vi "draw.vi"(0 "reference":refnum<class "ArrowHead.lvclass">, 1 "graphics":refnum<class "Graphics.lvclass">, 2 "p1":T1 {"y" format="%.2f"; "x" format="%.2f"}, 3 "p2":T1 {"y" format="%.2f"; "x" format="%.2f"}, 5 "error in (no error)":errorcluster) -> (14 "reference out":refnum<class "ArrowHead.lvclass">, 19 "error out":errorcluster)   [LabVIEW 2012, in "ArrowHead.lvclass"]
doc: "public void draw(Graphics2D g2, Point2D p, Point2D q)"
uses:
  <resource>/Framework/Providers/Open_GDS/UML/ArrowHead_class/ArrowHead.lvclass
  <resource>/Framework/Providers/Open_GDS/UML/Graphics_class/Graphics.lvclass
  <resource>/Framework/Providers/Open_GDS/UML/General/Point/Point Point2D.ctl
  <resource>/Framework/Providers/Open_GDS/UML/ArrowHead_class/ArrowHead.lvclass/ArrowHead.ctl
  <resource>/Framework/Providers/Open_GDS/UML/ArrowHead_class/ArrowHeadType.ctl
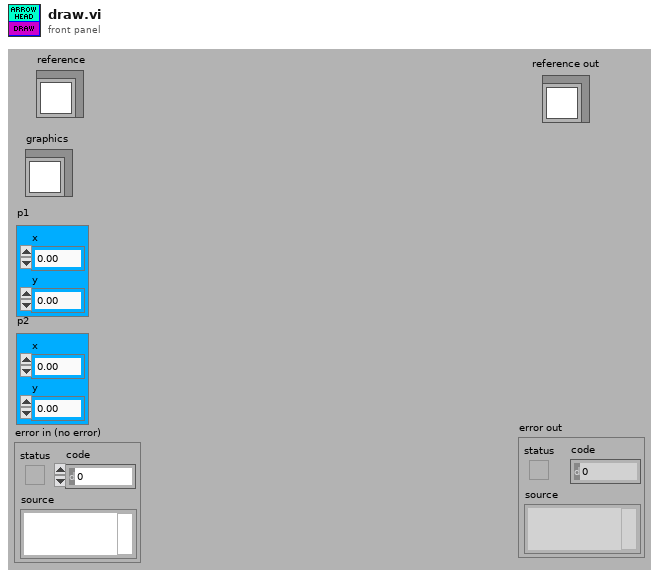
[diagram p1: front panel]
types:
  T1 = typedef "Point Point2D.ctl" = cluster{"x":dbl, "y":dbl}
  T2 = typedef "ArrowHead.lvclass/ArrowHeadType.ctl" = enum16{"NONE", "TRIANGLE", "BLACK_TRIANGLE", "V", "HALF_V", "DIAMOND", "BLACK_DIAMOND"}
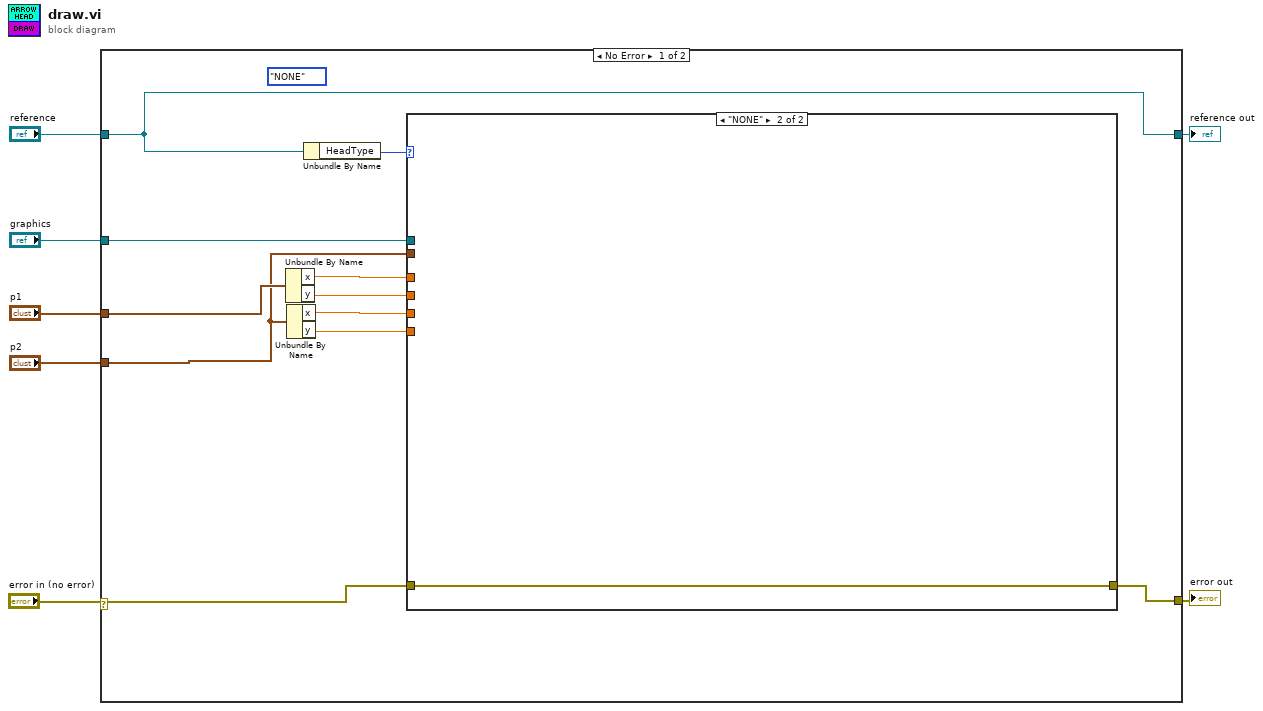
[diagram p0: block diagram]
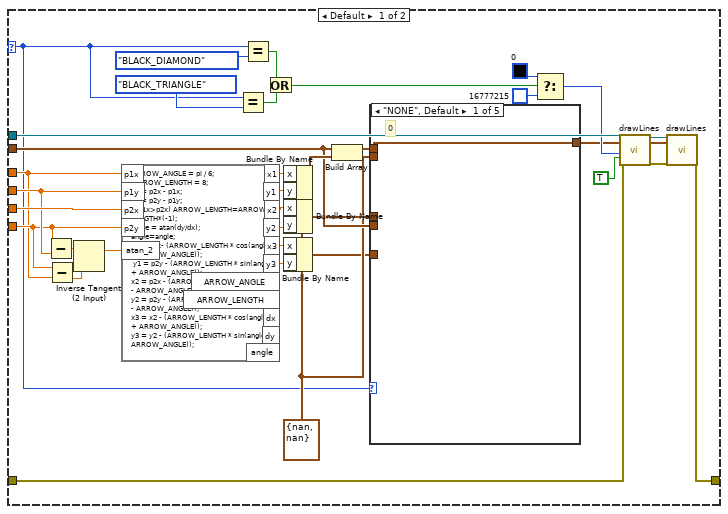
[diagram p2: hidden frame]
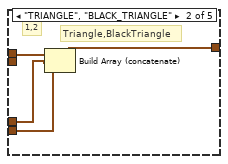
[diagram p3: hidden frame]
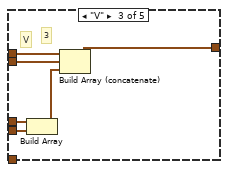
[diagram p4: hidden frame]
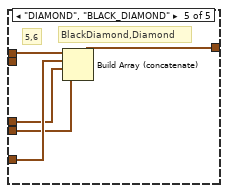
[diagram p6: hidden frame]
diagram:
  n1 = case shown="No Error" "error in (no error)" {
    selector: "error in (no error)" -> [w9 w72]
    tunnel: "reference" -> [w8 w73]
    tunnel: [w18 w72] -> w6
    tunnel: [w8 w73] -> w5
    tunnel: "graphics" -> [w17 _]
    tunnel: "p1" -> [w16 _]
    tunnel: "p2" -> [w15 _]
    frame No Error {
      (unwired) ArrowHeadType."NONE" ("HeadType")
      n2 = Unbundle By Name(w16) -> ("x"=w14:dbl, "y"=w13:dbl)
      n3 = Unbundle By Name(w15) -> ("x"=w12:dbl, "y"=w11:dbl)
      n4 = Unbundle By Name(w8) -> ("HeadType"=w10:T2)
      n5 = case shown="\"NONE\"" w10 {
        selector: w10 -> [w19 _]
        tunnel: w9 -> [w43 w71]
        tunnel: [w23 w71] -> w18
        tunnel: w17 -> [w53 _]
        tunnel: w14 -> [w27 _]
        tunnel: w13 -> [w30 _]
        tunnel: w12 -> [w47 _]
        tunnel: w11 -> [w28 _]
        tunnel: w15 -> [w39 _]
        frame Default {
          w37 = T1 {"x"=nan, "y"=nan} ("p1")
          n6 = Subtract(x=w28, y=w30) -> (x-y=w31:dbl)
          n7 = Subtract(x=w28, y=w27) -> (x-y=w29:dbl)
          n8 = Inverse Tangent (2 Input)(1:w29, 2:w31) -> (0:w32:dbl)
          n9 = formula code="ARROW_ANGLE = pi / 6;\n ARROW_LENGTH = 8;\ndx = p2x - p1x;\ndy = p2y - p1y;\nif(p1x>p2x) ARROW_LENGTH=ARROW_LENGTH*(-1);\nangle = atan(dy/dx);\nangle=angle;\nx1 = p2x- (ARROW_LENGTH * cos(angle + ARROW_ANGLE));\n y1 = p2y - (ARROW_LENGTH * sin(angle + ARROW_ANGLE));\nx2 = p2x - (ARROW_LENGTH * cos(angle - ARROW_ANGLE));\ny2 = p2y - (ARROW_LENGTH * sin(angle - ARROW_ANGLE));\nx3 = x2 - (ARROW_LENGTH * cos(angle + ARROW_ANGLE));\ny3 = y2 - (ARROW_LENGTH * sin(angle + ARROW_ANGLE));"("p1x"=w27, "p1y"=w30, "p2x"=w47, "p2y"=w28, "atan_2"=w32) -> ("x1"=w46:dbl, "y1"=w45:dbl, "x2"=w41:dbl, "y2"=w40:dbl, "x3"=w36:dbl, "y3"=w35:dbl)  [unwired: 5 out]
          n10 = Equal?(x=w19, y=ArrowHeadType."BLACK_TRIANGLE") -> (x = y?=w49:bool)
          n11 = Equal?(x=w19, y=ArrowHeadType."BLACK_DIAMOND") -> (x = y?=w21:bool)
          n12 = Or(x=w21, y=w49) -> (x .or. y?=w33:bool)
          n13 = Bundle By Name(cluster=w37, "x"=w46, "y"=w45) -> (w44:T1)
          n14 = Bundle By Name(cluster=w37, "x"=w41, "y"=w40) -> (w38:T1)
          n15 = Bundle By Name(cluster=w37, "x"=w36, "y"=w35) -> (w34:T1)
          n16 = Build Array(w39, w44) -> (w42:T1[])
          n17 = case shown="\"NONE\", Default" w19 {
            tunnel: w42 -> [w54 w58 w64 w65 w70]
            tunnel: w37 -> [_ _ w63 _ _]
            tunnel: w38 -> [_ w57 w61 _ w68]
            tunnel: w39 -> [_ w55 w60 _ w66]
            tunnel: w34 -> [_ _ _ _ w69]
            tunnel: [w54 w56 w59 w65 w67] -> w25
            frame "NONE", Default {
              # "0"
            }
            frame "TRIANGLE", "BLACK_TRIANGLE" {
              # "1,2"
              # "Triangle,BlackTriangle"
              n18 = Build Array (concatenate)(w58, w57, w55) -> (w56:T1[])
            }
            frame "V" {
              # "3"
              # "V"
              n19 = Build Array(w61, w60) -> (w62:T1[])
              n20 = Build Array (concatenate)(w64, w63, w62) -> (w59:T1[])
            }
            frame "HALF_V" {
              # "4"
              # "HALF-V"
            }
            frame "DIAMOND", "BLACK_DIAMOND" {
              # "5,6"
              # "BlackDiamond,Diamond"
              n21 = Build Array (concatenate)(w70, w69, w68, w66) -> (w67:T1[])
            }
          }
          n22 = Select(t=u32 0, s=w33, f=u32 16777215) -> (s? t:f=w48:u32)
          n23 = call <resource>:"drawLines.vi"("reference"=w53, "points"=w25, "color(if not used=default color)"=w48, "fill?(F)"=TRUE, "error in (no error)"=w43) -> ("reference out"=w26:refnum<class "Graphics.lvclass">, "error out"=w24:errorcluster)  [unwired: 2 in, 11 out]
          n24 = call <resource>:"drawLines.vi"("reference"=w26, "points"=w25, "error in (no error)"=w24) -> ("error out"=w23:errorcluster)  [unwired: 4 in, 12 out]
        }
        frame "NONE" {
        }
      }
    }
    frame Error {
    }
  }
  "reference out" <- w5
  "error out" <- w6
